vi "Teleop.vi"(10 "Match Info":T1={"Autonomous Elapsed Seconds"=0.0, "TeleOp Elapsed Seconds"=0.0, "Disabled Elapsed Seconds"=0.0, "Visited Autonomous"=FALSE, "Visited TeleOp"=FALSE, "Visited Disabled"=FALSE, "Autonomous Settings"={"Autonomous Style"=enum."Independent", "VI Refnum"=refnum}}, 11 "Call Context":T2) -> ()   [LabVIEW 2015]
doc: "This VI is called for each TeleOp packet received from the DS where the robot is not disabled. It is often used to read from the joysticks and update I/O or to update setpoints for timed control loops. It should complete and return within 20 milliseconds or it may miss DS packets."
uses:
  <vilib>/Rock Robotics/WPI/DriverStation/WPI_DriverStationDerivedRobotMode.ctl
  <vilib>/Rock Robotics/WPI/DriverStation/WPI_DriverStationMatch Info.ctl
  <userlib>/836-Library/Drive/Drive Code/Drive Code Support/Drive Code Bundle.ctl
  <userlib>/836-Library/Drive/Drive Code/Drive Code Support/Sensor Cluster.ctl
  <userlib>/836-Library/Drive/Drive Code/Drive Code Support/Camera Cluster.ctl
  <userlib>/836-Library/Drive/Drive Code/Drive Code Support/Drive Code Notifier.ctl
  <userlib>/836-Library/Drive/Drive Code/Drive Code Support/Drive Code Command.ctl
  <userlib>/836-Library/Pneumatics/Support Code/Pneumatics Command.ctl
  <vilib>/Rock Robotics/WPI/Utilities/WPI_GetSetVariantRefNum.vi
  <userlib>/836-Library/Pneumatics/Support Code/Pneumatics Command Set Tele.vi
  <userlib>/836-Library/Drive/Drive Code/Drive Code Support/Drive Loop Cheesey Drive.vi
  Pneumatic Commands.ctl
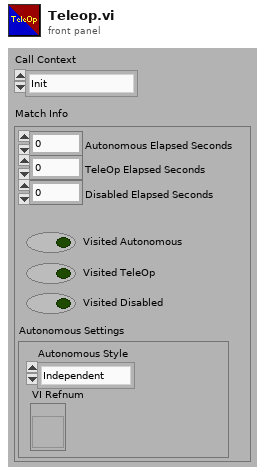
[diagram p1: front panel]
types:
  T1 = typedef "WPI_DriverStationMatch Info.ctl" = cluster{"Autonomous Elapsed Seconds":dbl, "TeleOp Elapsed Seconds":dbl, "Disabled Elapsed Seconds":dbl, "Visited Autonomous":bool, "Visited TeleOp":bool, "Visited Disabled":bool, "Autonomous Settings":cluster{"Autonomous Style":enum16{"Iterative", "Independent"}, "VI Refnum":refnum<vi>}}
  T2 = typedef "WPI_DriverStationDerivedRobotMode.ctl" = enum16{"Init", "Execute", "Stop"}
  T3 = typedef "Drive Code Bundle.ctl" = cluster{"Sensor Data":T4, "Drive Command rt fifo":refnum<k33>}
  T4 = typedef "Sensor Cluster.ctl" = cluster{"Gyro Data":cluster{"Gyro RT FIFO":refnum<k33>, "Gyro Current":dbl, "Gyro Hold":dbl}, "Encoder Data":cluster{"Encoder RT FIFO":refnum<k33>, "Encoder Current":dbl, "Encoder Hold":dbl}, "Camera Data":cluster{"Camera RT FIFO":refnum<k33>, "Camera Current":T5}}
  T5 = typedef "Camera Cluster.ctl" = cluster{" Angle":dbl, "Valid":bool}
  T6 = typedef "WPI_JoystickDevRef.ctl" = cluster{"Device":T7}
  T7 = typedef "WPI_JoystickDeviceEnum.ctl" = enum16{"USB 0", "USB 1", "USB 2", "USB 3", "USB 4", "USB 5"}
  T8 = typedef "Pneumatic Commands.ctl" = enum16{"Go Up", "Go Down", "Nothing"}
  T9 = typedef "Pneumatics Command.ctl" = enum16{"Nothing", "Forward", "Reverse", "Toggle"}
  T10 = typedef "WPI_MotorControlDeviceRef.ctl" = cluster{"DeviceStatus":errorcluster, "Type":T11, "PWM":cluster{"PWM Channel":T12, "DeadBand":T13}, "CAN":cluster{"Device Number":u8, "Control Mode":T14, "Semaphore":T15, "Max Vout":dbl, "TalonSRX Control Mode":T16}, "Invert":bool}
  T11 = typedef "WPI_MotorControlType.ctl" = enum16{"PWM", "CAN", "CANTalonSRX"}
  T12 = typedef "FPGA_DIOPWMChannel.ctl" = enum8{"PWM 0", "PWM 1", "PWM 2", "PWM 3", "PWM 4", "PWM 5", "PWM 6", "PWM 7", "PWM 8", "PWM 9", "PWM MXP 0", "PWM MXP 1", "PWM MXP 2", "PWM MXP 3", "PWM MXP 4", "PWM MXP 5", "PWM MXP 6", "PWM MXP 7", "PWM MXP 8", "PWM MXP 9", "Invalid"}
  T13 = typedef "WPI_PWMDeadband.ctl" = cluster{"Name":string, "maxPositivePwm":i32, "minPositivePwm":i32, "centerPwm":i32, "maxNegativePwm":i32, "minNegativePwm":i32, "angularRange":u16}
  T14 = typedef "WPI_CANJaguar_ControlMode.ctl" = enum8{"Percent VBus", "Current", "Speed", "Position", "Voltage"}
  T15 = typedef "Semaphore RefNum" = refnum<k1>
  T16 = typedef "WPI_CANTalonSRX_APIControlMode.ctl" = enum8{"Percent VBus", "Speed", "Position", "Slave", "Unchanged / Invalid", "Voltage Compensation", "Current", "Motion Profile"}
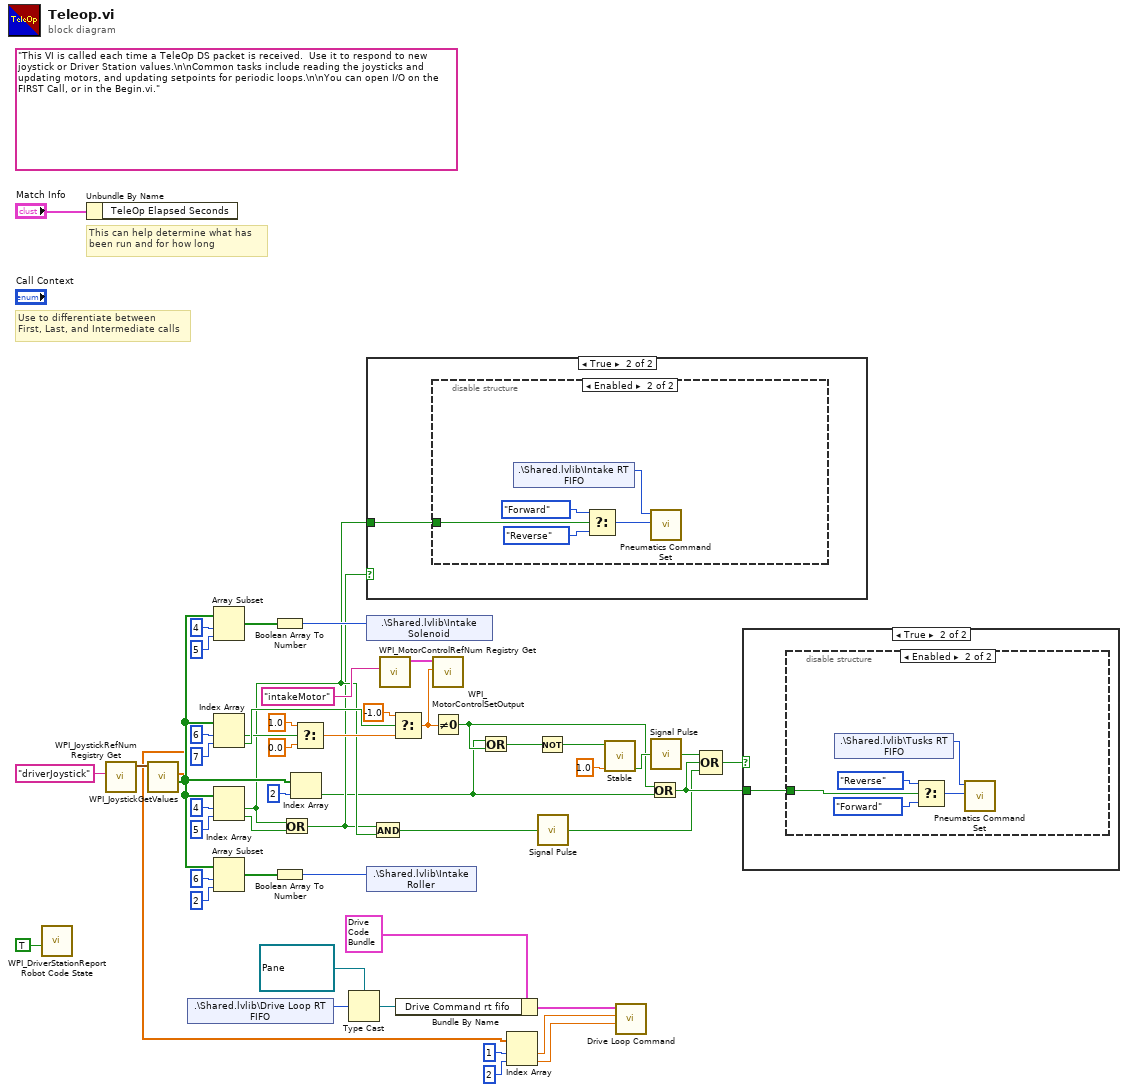
[diagram p0: block diagram]
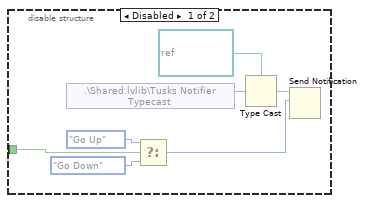
[diagram p3: hidden frame]
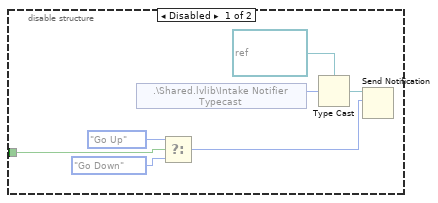
[diagram p5: hidden frame]
diagram:
  (unwired) "This VI is called each time a TeleOp DS packet is received.  Use it to respond to new joystick or Driver Station values.\n\nCommon tasks include reading the joysticks and updating motors, and updating setpoints for periodic loops.\n\nYou can open I/O on the FIRST Call, or in the Begin.vi."
  # "Use to differentiate between\nFirst, Last, and Intermediate calls"
  # "This can help determine what has\nbeen run and for how long"
  n1 = call <vilib>:"WPI_DriverStationReport Robot Code State.vi"("TeleOp"=TRUE ("Autonomous")) -> ()  [unwired: 10 in, 1 out]
  n2 = Unbundle By Name("Match Info") -> ()  [unwired: 1 out]
  n3 = call <vilib>:"WPI_JoystickRefNum Registry Get.vi"("refnum name"="driverJoystick") -> ("JoystickDevRef"=w46:T6)  [unwired: 1 in, 9 out]
  n4 = call <vilib>:"WPI_JoystickGetValues.vi"("JoystickDevRef"=w46) -> ("Buttons"=w26:bool[], "Axes"=w5:dbl[])  [unwired: 6 in, 3 out]
  n5 = shared-variable ".\\Shared.lvlib\\Drive Loop RT FIFO"() -> (w7:u32)  [unwired: 1 in, 1 out]
  n6 = Array Subset(array=w26, index=4, length=5) -> (w31:bool[])
  n7 = Index Array(array=w26, index #1=6 ("index"), index #2=7 ("index")) -> (element #1=w44:bool, element #2=w45:bool)
  n8 = Index Array(array=w26, index #1=4 ("index"), index #2=5 ("index")) -> (element #1=w23:bool, element #2=w47:bool)
  n9 = Array Subset(array=w26, index=6, length=2) -> (w32:bool[])
  n10 = Boolean Array To Number(Boolean array=w31) -> (number=w28:u32)
  n11 = Boolean Array To Number(Boolean array=w32) -> (number=w27:u32)
  n12 = Or(x=w23, y=w47) -> (x .or. y?=w22:bool)
  n13 = Index Array(array=w26, index=2) -> (element=w11:bool)
  n14 = Select(t=1.0, s=w44, f=0.0) -> (s? t:f=w42:dbl)
  n15 = Type Cast(type=refnum<k33> refnum ("Drive Command rt fifo"), x=w7) -> (*(type *) &x=w6:refnum<k33>)
  n16 = case shown="True" w22 {
    tunnel: w23 -> [_ w52]
    frame False {
    }
    frame True {
      n17 = disable-structure shown="Enabled" {
        disable-tunnel: w52 -> [w56 w62]
        frame Disabled {
          w55 = refnum<notifier> refnum items=["Go Up", "Go Down", "Nothing"] ("notifier out")
          n18 = shared-variable ".\\Shared.lvlib\\Intake Notifier Typecast"() -> (w54:u32)  [unwired: 1 in, 1 out]
          n19 = Select(t=Pneumatic_Commands."Go Up", s=w56, f=Pneumatic_Commands."Go Down") -> (s? t:f=w57:T8)
          n20 = Type Cast(type=w55, x=w54) -> (*(type *) &x=w53:refnum<notifier>)
          n21 = Send Notification(notification=w57, notifier=w53) -> ()  [unwired: 1 in, 2 out]
        }
        frame Enabled {
          n22 = shared-variable ".\\Shared.lvlib\\Intake RT FIFO"() -> (w60:u64)  [unwired: 1 in, 1 out]
          n23 = Select(t=Pneumatics_Command."Forward" ("Solenoid Command"), s=w62, f=Pneumatics_Command."Reverse" ("Solenoid Command")) -> (s? t:f=w61:T9)
          n24 = call-poly <userlib>:"Pneumatics Command Set.vi"("Solenoid Command"=w61, "RT FIFO"=w60) -> ()  [unwired: 9 in, 1 out]
        }
      }
    }
  }
  n25 = shared-variable ".\\Shared.lvlib\\Intake Solenoid"(w28) -> ()  [unwired: 1 in, 1 out]
  n26 = shared-variable ".\\Shared.lvlib\\Intake Roller"(w27) -> ()  [unwired: 1 in, 1 out]
  n27 = And(x=w22, y=w23) -> (x .and. y?=w21:bool)
  n28 = call <vilib>:"WPI_MotorControlRefNum Registry Get.vi"("refnum name"="intakeMotor") -> ("MotorControlDevRef"=w36:T10)  [unwired: 9 in, 1 out]
  n29 = Select(t=-1.0 ("f"), s=w45, f=w42) -> (s? t:f=w25:dbl)
  n30 = Bundle By Name(cluster=T3 {"Sensor Data"={"Gyro Data"={"Gyro RT FIFO"=refnum, "Gyro Current"=0.0, "Gyro Hold"=0.0}, "Encoder Data"={"Encoder RT FIFO"=refnum, "Encoder Current"=0.0, "Encoder Hold"=0.0}, "Camera Data"={"Camera RT FIFO"=refnum, "Camera Current"={" Angle"=0.0, "Valid"=FALSE}}}, "Drive Command rt fifo"=refnum} ("Drive Loop Cluster"), "Drive Command rt fifo"=w6) -> (w9:T3)
  n31 = call <vilib>:"WPI_MotorControlSetOutput.vi"("Output"=w25, "MotorControlDevRef"=w36) -> ()  [unwired: 7 in, 3 out]
  n32 = Not Equal To 0?(x=w25) -> (x != 0?=w14:bool)
  n33 = Or(x=w11, y=w14) -> (x .or. y?=w13:bool)
  n34 = Index Array(array=w5, index #1=1 ("index"), index #2=2 ("index")) -> (element #1=w2:dbl, element #2=w1:dbl)
  n35 = Not(x=w13) -> (.not. x?=w15:bool)
  n36 = call <userlib>:"Signal Pulse.vi"("Input"=w21) -> ("Output"=w12:bool)
  n37 = call <userlib>:"Stable.vi"("Eval Period (sec)"=1.0, "Signal Input"=w15) -> ("Stable"=w18:bool)  [unwired: 9 in]
  n38 = call-poly <userlib>:"Drive Loop Command.vi"("Wheel"=w1, "Throttle"=w2, "Drive Loop Cluster"=w9) -> ()  [unwired: 9 in]
  n39 = Or(x=w14, y=w11) -> (x .or. y?=w19:bool)
  n40 = call <userlib>:"Signal Pulse.vi"("Input"=w18) -> ("Output"=w16:bool)
  n41 = Compound Arithmetic op=OR(w16, w19, w12) -> (w20:bool)
  n42 = case shown="True" w20 {
    tunnel: w19 -> [_ w65]
    frame False {
    }
    frame True {
      n43 = disable-structure shown="Enabled" {
        disable-tunnel: w65 -> [w66 w74]
        frame Disabled {
          w69 = refnum<notifier> refnum items=["Go Up", "Go Down", "Nothing"] ("notifier out")
          n44 = shared-variable ".\\Shared.lvlib\\Tusks Notifier Typecast"() -> (w67:u32)  [unwired: 1 in, 1 out]
          n45 = Select(t=Pneumatic_Commands."Go Up", s=w66, f=Pneumatic_Commands."Go Down") -> (s? t:f=w70:T8)
          n46 = Type Cast(type=w69, x=w67) -> (*(type *) &x=w68:refnum<notifier>)
          n47 = Send Notification(notification=w70, notifier=w68) -> ()  [unwired: 1 in, 2 out]
        }
        frame Enabled {
          n48 = shared-variable ".\\Shared.lvlib\\Tusks RT FIFO"() -> (w73:u64)  [unwired: 1 in, 1 out]
          n49 = Select(t=Pneumatics_Command."Reverse" ("Solenoid Command"), s=w74, f=Pneumatics_Command."Forward" ("Solenoid Command")) -> (s? t:f=w77:T9)
          n50 = call-poly <userlib>:"Pneumatics Command Set.vi"("Solenoid Command"=w77, "RT FIFO"=w73) -> ()  [unwired: 9 in, 1 out]
        }
      }
    }
  }
